vi "important information-autoConn1.vi"() -> ()   [LabVIEW 2011]
doc: "ID=0x6007"
panel:
  in  "ok":bool
  out "tip":string="    当前已启用【USB掉线重启】功能，系统会自动以上一次配置启动设备。\n    主要应用于工业环境，提高可靠性，保证CAN调试器不间断运行。\n    系统不再弹出配置对话框，若要更改配置，请在\"设备操作”菜单中，关闭设备，再启动设备。" caption="Important:"
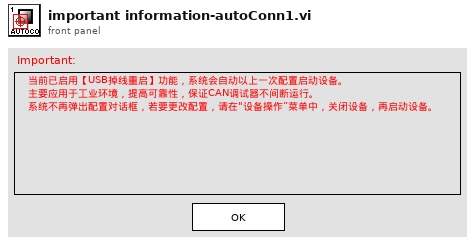
[diagram p1: front panel]
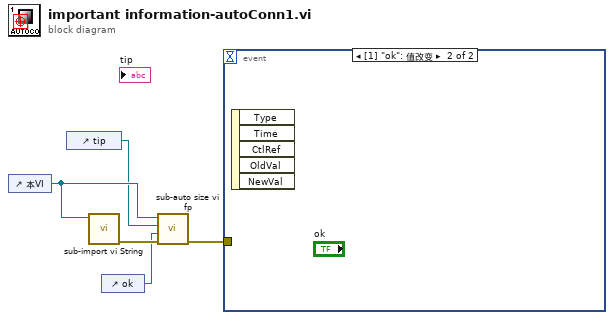
[diagram p0: block diagram]
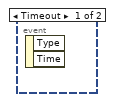
[diagram p2: hidden frame]
diagram:
  n1 = control-ref of="本VI"() -> (w3:refnum<vi>)
  n2 = control-ref of="tip"() -> (w2:refnum<vi>)
  n3 = call "sub-import vi String.vi"("vi ref"=w3) -> ("error out"=w5:errorcluster)  [unwired: 10 in]
  n4 = control-ref of="ok"() -> (w1:refnum<vi>)
  n5 = call "sub-auto size vi fp.vi"("error in (no error)"=w5, "btn ref"=w1, "str ref"=w2, "vi ref"=w3) -> ("error out"=w4:errorcluster)  [unwired: 7 in]
  n6 = event shown="[1] \"ok\": 值改变" {
    selector: _ -> [_ _]
    dyn-events: _ -> [_ _]
    timeout: _ -> [_ _]
    tunnel: w4 -> [_ _]
    event Timeout {
      n7 = event-data() -> ()  [unwired: 1 in, 2 out]
    }
    event "ok": Value Change {
      n8 = event-data() -> ()  [unwired: 1 in, 5 out]
    }
  }
